vi "String Not Included.vi"() -> ()   [LabVIEW 2017, in "Assertions.Tests.lvlib" / "Assert Error Message Contains String.lvlib"]
uses:
  Assert Error Message Contains String.lvlib
  e8b37827-c40c-4938-b4cd-332d526e978e.vi
  <vilib>/Utility/error.llb/Error Cluster From Error Code.vi
  src/Transparent Assertions/Constraints/IsEqual/Create.vi
  <vilib>/ErrorRing/Error Ring.xnode
  src/Transparent Assertions/Constraints/IsEqual/IsEqual.lvclass
  src/Transparent Assertions/Assertions/Assertions.lvlib
  Assertions.Tests.lvlib
panel:
  out "error out":errorcluster
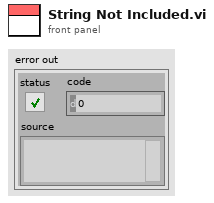
[diagram p1: front panel]
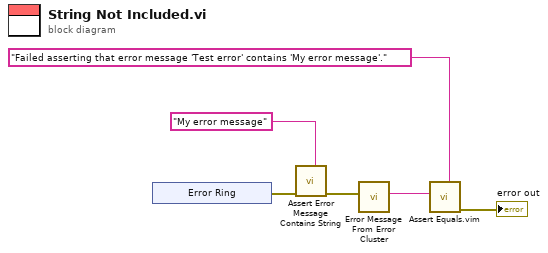
[diagram p0: block diagram]
diagram:
  n1 = xnode "Error Ring"() -> ("error out"=w3:errorcluster)
  n2 = call "Assert Error Message Contains String.vi"("Expected"="My error message", "error in (no error)"=w3) -> ("error out"=w2:errorcluster)  [unwired: 9 in]
  n3 = call "Error Message From Error Cluster.vi"("Error"=w2) -> ("Error Message"=w5:string)  [unwired: 10 in]
  n4 = call "Assert Equals.vim"("Expected"="Failed asserting that error message 'Test error' contains 'My error message'." ("Needle"), "Actual"=w5) -> ("error out"=→"error out":errorcluster)  [unwired: 9 in]
